vi "undock.vi"(8 "error in (no error)":errorcluster, 9 "undock?":T1, 10 "VI path":path, 11 "component in":refnum<class "GenericToplevelComponent.lvclass">) -> (0 "error out":errorcluster, 3 "component out":refnum<class "GenericToplevelComponent.lvclass">)   [LabVIEW 2011, in "GenericToplevelComponent.lvclass"]
uses:
  GenericToplevelComponent.lvclass
  main/labview_source/controls/undock_button.ctl
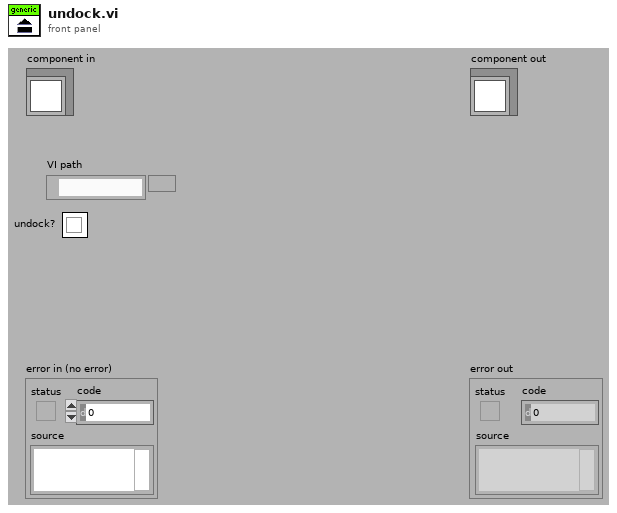
[diagram p1: front panel]
types:
  T1 = typedef "undock_button.ctl" = bool
  T2 = enum32{"Invalid", "Standard", "Closed", "Hidden", "Minimized", "Maximized"}
  T3 = typedef "controls_refs.ctl" = cluster{"buttons":cluster{"start_focus":refnum<vi>, "start_single_sweep":refnum<vi>, "start_experiment":refnum<vi>, "save":refnum<vi>, "exit":refnum<vi>}, "tabs":cluster{"main":refnum<vi>, "settings":refnum<vi>}, "subpanels":cluster{"imagingMode":refnum<vi>, "scanHead":refnum<vi>, "display":refnum<vi>, "experimentController":refnum<vi>, "instrument":refnum<vi>, "stage":refnum<vi>, "stimulator":refnum<vi>, "dataCollection":refnum<vi>, "analyser":refnum<vi>, "daq":refnum<vi>, "imageAssembler":refnum<vi>}, "drop-downs":cluster{"imagingMode":refnum<vi>, "experimentalController":refnum<vi>, "objective":refnum<vi>}, "status lights":cluster{"experimentController":refnum<vi>, "imagingMode":refnum<vi>, "scanHead":refnum<vi>, "daq":refnum<vi>, "imageAssembler":refnum<vi>, "dataCollection":refnum<vi>, "display":refnum<vi>, "analyser":refnum<vi>, "stage":refnum<vi>, "stimulator":refnum<vi>, "instrument":refnum<vi>}, "message":refnum<vi>, "stimulator enabled?":refnum<vi>, "saving":cluster{"data folder path":refnum<vi>, "file base name":refnum<vi>, "notebook":refnum<vi>}, "progress bar":refnum<vi>, "update icon":refnum<vi>, "title":refnum<vi>, "main vi":refnum<vi>, "user":refnum<vi>}
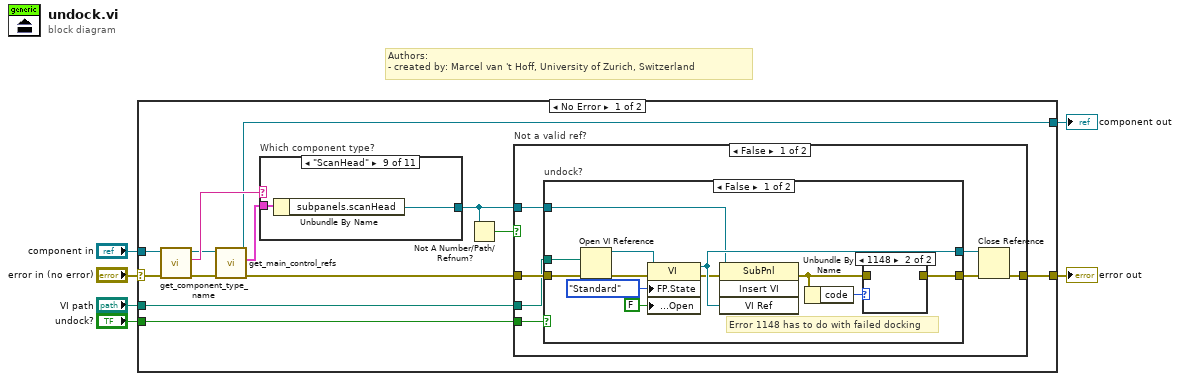
[diagram p0: block diagram]
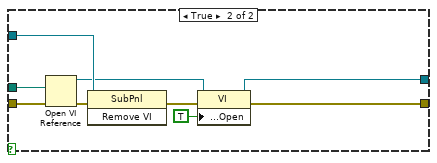
[diagram p3: hidden frame]
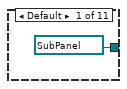
[diagram p5: hidden frame]
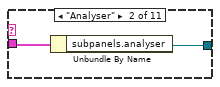
[diagram p6: hidden frame]
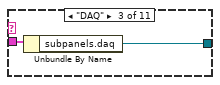
[diagram p7: hidden frame]
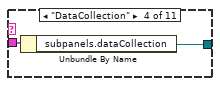
[diagram p8: hidden frame]
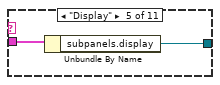
[diagram p9: hidden frame]
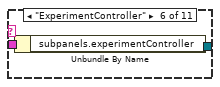
[diagram p10: hidden frame]
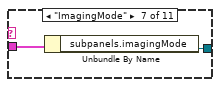
[diagram p11: hidden frame]
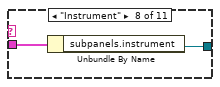
[diagram p12: hidden frame]
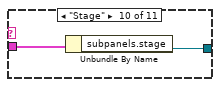
[diagram p13: hidden frame]
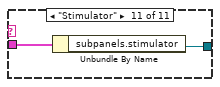
[diagram p14: hidden frame]
diagram:
  # "Authors: \n- created by: Marcel van 't Hoff, University of Zurich, Switzerland"
  n1 = case shown="No Error" "error in (no error)" {
    selector: "error in (no error)" -> [w13 w72]
    tunnel: [w10 w72] -> w5
    tunnel: [w15 w71] -> w3
    tunnel: "component in" -> [w16 w71]
    tunnel: "undock?" -> [w8 _]
    tunnel: "VI path" -> [w7 _]
    frame No Error {
      n2 = call-dynamic "get_component_type_name.vi"("error in (no error)"=w13, "GenericPlugin in"=w16) -> ("error out"=w14:errorcluster, "component type"=w19:string, "GenericPlugin out"=w18:refnum<class "GenericToplevelComponent.lvclass">)  [unwired: 7 in]
      n3 = call-dynamic "get_main_control_refs.vi"("error in (no error)"=w14, "GenericPlugin.lvclass in"=w18) -> ("error out"=w11:errorcluster, "control references"=w17:T3, "GenericPlugin.lvclass out"=w15:refnum<class "GenericToplevelComponent.lvclass">)  [unwired: 7 out]
      n4 = case "Which component type?" shown="\"ScanHead\"" w19 {
        tunnel: w17 -> [_ w52 w54 w55 w58 w60 w62 w64 w66 w68 w70]
        tunnel: [refnum<vi> refnum ("stimulator") w51 w53 w56 w57 w59 w61 w63 w65 w67 w69] -> w9
        frame Default {
        }
        frame "Analyser" {
          n5 = Unbundle By Name(w52) -> ("subpanels.analyser"=w51:refnum<vi>)
        }
        frame "DAQ" {
          n6 = Unbundle By Name(w54) -> ("subpanels.daq"=w53:refnum<vi>)
        }
        frame "DataCollection" {
          n7 = Unbundle By Name(w55) -> ("subpanels.dataCollection"=w56:refnum<vi>)
        }
        frame "Display" {
          n8 = Unbundle By Name(w58) -> ("subpanels.display"=w57:refnum<vi>)
        }
        frame "ExperimentController" {
          n9 = Unbundle By Name(w60) -> ("subpanels.experimentController"=w59:refnum<vi>)
        }
        frame "ImagingMode" {
          n10 = Unbundle By Name(w62) -> ("subpanels.imagingMode"=w61:refnum<vi>)
        }
        frame "Instrument" {
          n11 = Unbundle By Name(w64) -> ("subpanels.instrument"=w63:refnum<vi>)
        }
        frame "ScanHead" {
          n12 = Unbundle By Name(w66) -> ("subpanels.scanHead"=w65:refnum<vi>)
        }
        frame "Stage" {
          n13 = Unbundle By Name(w68) -> ("subpanels.stage"=w67:refnum<vi>)
        }
        frame "Stimulator" {
          n14 = Unbundle By Name(w70) -> ("subpanels.stimulator"=w69:refnum<vi>)
        }
      }
      n15 = Not A Number/Path/Refnum?(number/path/refnum=w9) -> (NaN/Path/Refnum?=w12:bool)
      n16 = case "Not a valid ref?" shown="False" w12 {
        tunnel: w11 -> [w25 w49]
        tunnel: [w22 w49] -> w10
        tunnel: w9 -> [w24 _]
        tunnel: w8 -> [w26 _]
        tunnel: w7 -> [w23 _]
        frame False {
          n17 = case "undock?" shown="False" w26 {
            tunnel: w25 -> [w38 w44]
            tunnel: w23 -> [w37 w42]
            tunnel: [w27 w46] -> w21
            tunnel: w24 -> [w35 w45]
            tunnel: [w36 w41] -> w20
            frame False {
              # "Error 1148 has to do with failed docking"
              n18 = Open VI Reference(vi path=w37, error in (no error)=w38) -> (vi reference=w30:refnum<vi>, error out=w31:errorcluster)  [unwired: 1 in, 3 out]
              n19 = property class="VI"(reference=w30, error in=w31, "FP.State"=T2."Standard" ("Front Panel Window:State"), "Front Panel.Open"=FALSE ("Front Panel Window:Open")) -> (reference out=w36:refnum<vi>, error out=w34:errorcluster)
              n20 = invoke class="SubPnl" method="Insert VI"(reference=w35, error in=w34, "VI Ref"=w36) -> (error out=w28:errorcluster)  [unwired: 1 in, 3 out]
              n21 = Unbundle By Name(w28) -> ("code"=w29:i32)
              n22 = case shown="1148" w29 {
                tunnel: [w39 _] -> w27
                tunnel: w28 -> [w39 _]
                frame Default {
                }
                frame 1148 {
                }
              }
            }
            frame True {
              n23 = Open VI Reference(vi path=w42, error in (no error)=w44) -> (vi reference=w40:refnum<vi>, error out=w43:errorcluster)  [unwired: 1 in, 3 out]
              n24 = invoke class="SubPnl" method="Remove VI"(reference=w45, error in=w43) -> (error out=w47:errorcluster)  [unwired: 1 in, 2 out]
              n25 = property class="VI"(reference=w40, error in=w47, "Front Panel.Open"=TRUE ("Front Panel Window:Open")) -> (reference out=w41:refnum<vi>, error out=w46:errorcluster)
            }
          }
          n26 = Close Reference(reference=w20, error in (no error)=w21) -> (error out=w22:errorcluster)
        }
        frame True {
        }
      }
    }
    frame Error {
    }
  }
  "error out" <- w5
  "component out" <- w3
